vi "lockin - add phase element.vi"(10 "Channels: Lockin":T1 {"REF phi (°)" format="%#_3g"}) -> (2 "Channels: Lockin Out":T1 {"REF phi (°)" format="%#_3g"})   [LabVIEW 2016]
uses:
  Instrument.Lockin/Typedefs/REF-cluster.ctl
  Instrument.Lockin/Typedefs/REF_f-array.ctl
  Instrument.Lockin/Typedefs/REF_phi-array.ctl
  Instrument.Lockin/Instrument.Lockin.lvclass
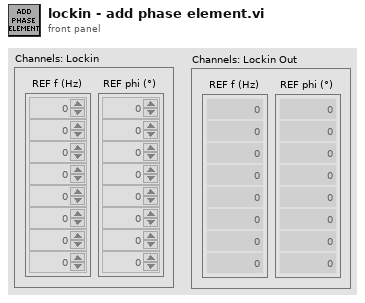
[diagram p1: front panel]
types:
  T1 = typedef "Instrument.Lockin.lvclass/REF-cluster.ctl" = cluster{"REF f (Hz)":T2, "REF phi (°)":T3}
  T2 = typedef "Instrument.Lockin.lvclass/REF_f-array.ctl" = dbl[]
  T3 = typedef "Instrument.Lockin.lvclass/REF_phi-array.ctl" = dbl[]
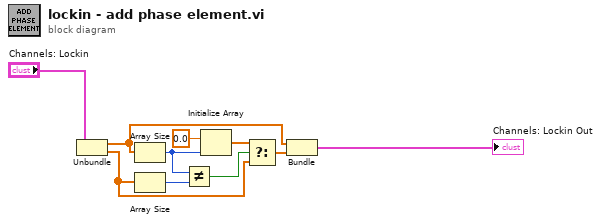
[diagram p0: block diagram]
diagram:
  n1 = Unbundle("Channels: Lockin") -> ("REF f (Hz)"=w6:T2, "REF phi (°)"=w4:T3)
  n2 = Array Size(array=w6) -> (size(s)=w1:i32)
  n3 = Array Size(array=w4) -> (size(s)=w7:i32)
  n4 = Not Equal?(x=w1, y=w7) -> (x != y?=w8:bool)
  n5 = Initialize Array(0.0 ("element"), w1) -> (w3:dbl[])
  n6 = Select(t=w3, s=w8, f=w4) -> (s? t:f=w5:T3)
  n7 = Bundle("REF f (Hz)"=w6, "REF phi (°)"=w5) -> (→"Channels: Lockin Out":cluster{"REF f (Hz)":T2, "REF phi (°)":T3})  [unwired: 1 in]
